vi "Get Interface.vi"(11 "Transceiver Thread in":refnum<class "Transceiver Thread.lvclass">) -> (2 "Interface":refnum<class "Transceiver Interface.lvclass">, 3 "Transceiver Thread out":refnum<class "Transceiver Thread.lvclass">)   [LabVIEW 2017, in "Data Sharing Framework Core.lvlib" / "Data Sharing Framework Engine.lvlib" / "Transceiver Thread.lvclass"]
uses:
  Transceiver Thread.lvclass
  Interfaces/Transceiver Interface/Transceiver Interface.lvclass
  Transceiver Thread.lvclass/Transceiver Thread.ctl
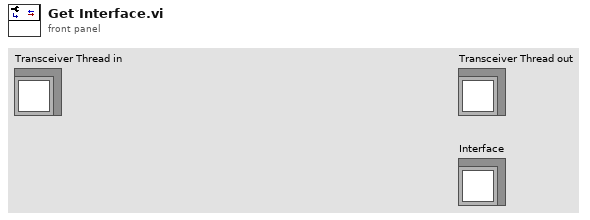
[diagram p1: front panel]
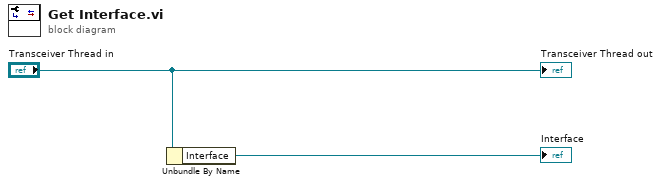
[diagram p0: block diagram]
diagram:
  n1 = Unbundle By Name("Transceiver Thread in") -> ("Interface"=→"Interface":refnum<class "Transceiver Interface.lvclass">)
  "Transceiver Thread out" <- "Transceiver Thread in"
